vi "BallShear_PackageAnalysis.vi"(8 "Original Image Path":path, 9 "Analyze":bool, 11 "Image Directory":path) -> (1 "Success":bool, 3 "Analyzed Image Path":path)   [LabVIEW 2013]
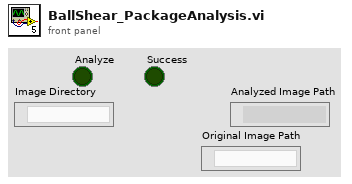
[diagram p1: front panel]
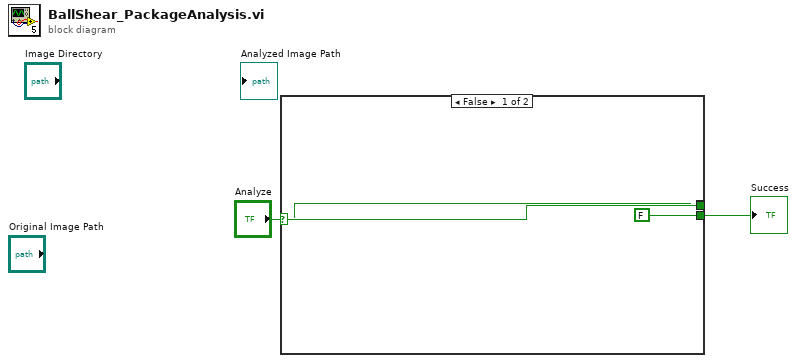
[diagram p0: block diagram]
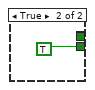
[diagram p2: hidden frame]
diagram:
  n1 = case shown="False" "Analyze" {
    selector: "Analyze" -> [w3 _]
    tunnel: [w3 w6] -> _
    tunnel: "Analyze" -> [_ w6]
    tunnel: [FALSE ("Power") TRUE ("Power")] -> w1
    frame False {
    }
    frame True {
    }
  }
  "Success" <- w1
